vi "FileIO-ReadWrite-FeatureList.vi"(0 "Filepath":path, 5 "Feature List (In)":T1(array[cluster]), 7 "Read/Write":enum16{"Read", "Write"}(ring), 11 "Error In":errorcluster) -> (4 "Feature List (Out)":T1(array[cluster]), 15 "Error Out":errorcluster)   [LabVIEW 2015]
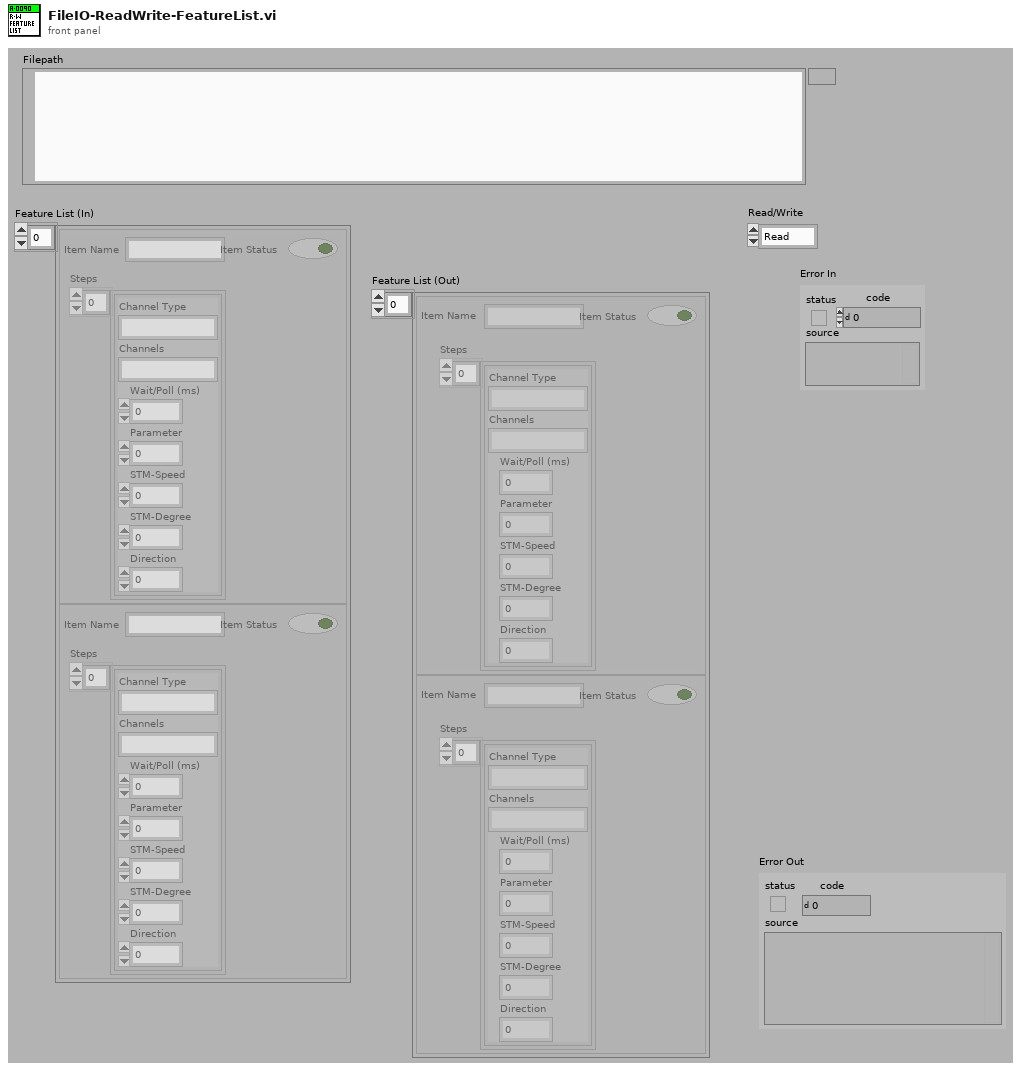
[diagram p1: front panel]
types:
  T1 = cluster{"Item Name":string, "Item Status":bool, "Steps":cluster{"Channel Type":string, "Channels":string, "Wait/Poll (ms)":u32, "Parameter":u8, "STM-Speed":i32, "STM-Degree":u32, "Direction":u8}[]}[]
  T2 = enum16{"read/write", "read-only", "write-only", "write-only (truncate)"}
  T3 = enum16{"open", "replace", "create", "open or create", "replace or create", "replace or create with confirmation"}
  T4 = cluster{"Item Name":string, "Item Status":bool, "Steps":cluster{"Channel Type":string, "Channels":string, "Wait/Poll (ms)":u32, "Parameter":u8, "STM-Speed":i32, "STM-Degree":u32, "Direction":u8}[]}
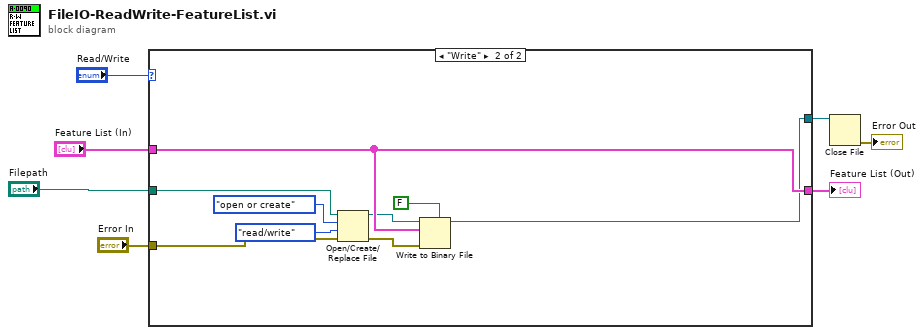
[diagram p0: block diagram]
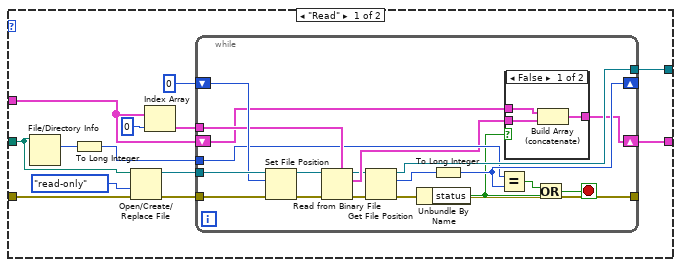
[diagram p2: hidden frame]
diagram:
  n1 = case shown="\"Write\"" "Read/Write" {
    tunnel: "Error In" -> [w20 w52]
    tunnel: "Filepath" -> [w14 w51]
    tunnel: [w9 w50] -> w4
    tunnel: "Feature List (In)" -> [w10 w50]
    tunnel: [w12 w47] -> w2
    frame "Read" {
      n2 = File/Directory Info(path=w14) -> (size=w8:i64)  [unwired: 1 in, 6 out]
      n3 = To Long Integer(number=w8) -> (32bit integer=w13:i32)
      n4 = Open/Create/Replace File(file path (use dialog)=w14, error in=w20, access (0:read/write)=T2."read-only" ("open mode (0)")) -> (refnum out=w18:refnum<file>, error out=w17:errorcluster)  [unwired: 3 in, 1 out]
      n5 = Index Array(array=w10, index=0) -> (element=w15:T4)
      n6 = while {
        tunnel: w18 -> [w39]
        tunnel: w17 -> [w38]
        tunnel: [w37] -> w12
        shift-right: [w34] -> _
        shift-left: 0 ("offset") -> [w36]
        tunnel: w15 -> [w35]
        tunnel: w13 -> [w33]
        shift-right: [w27] -> w9
        shift-left: w10 -> [w29]
        tunnel: [w21] -> _
        stop <- w31 stop-if-true
        n7 = Set File Position(offset (in bytes) (0)=w36, refnum=w39, error in=w38) -> (refnum out=w26:refnum<file>, error out=w25:errorcluster)  [unwired: 1 in]
        n8 = Read from Binary File(5:w35, 8:w25, 11:w26) -> (0:w23:errorcluster, 2:w28:T4, 3:w24:refnum<file>)  [unwired: 3 in, 1 out]
        n9 = Get File Position(4:w23, 7:w24) -> (0:w21:errorcluster, 2:w22:i64, 3:w37:refnum<file>)
        n10 = Unbundle By Name(w21) -> ("status"=w30:bool)
        n11 = To Long Integer(number=w22) -> (32bit integer=w34:i32)
        n12 = Equal?(x=w33, y=w34) -> (x = y?=w32:bool)
        n13 = case shown="False" w30 {
          tunnel: w29 -> [w42 w43]
          tunnel: w28 -> [w41 _]
          tunnel: [w40 w43] -> w27
          frame False {
            n14 = Build Array (concatenate)(w42, w41) -> (w40:T1)
          }
          frame True {
          }
        }
        n15 = Or(x=w32, y=w30) -> (x .or. y?=w31:bool)
      }
    }
    frame "Write" {
      n16 = Open/Create/Replace File(file path (use dialog)=w51, error in=w52, operation (0:open)=T3."open or create", access (0:read/write)=enum16{"read/write", "read-only", "write-only"}."read/write") -> (refnum out=w49:refnum<file>, error out=w48:errorcluster)  [unwired: 2 in, 1 out]
      n17 = Write to Binary File(file (use dialog)=w49, data=w50, error in=w48, 5:FALSE ("prepend array or string size? (T)")) -> (refnum out=w47:refnum<file>)  [unwired: 2 in, 2 out]
    }
  }
  "Feature List (Out)" <- w4
  n18 = Close File(refnum=w2) -> (error out=→"Error Out":errorcluster)  [unwired: 1 in, 1 out]
